vi "Bool_array_to_digital_waveform.vi"(0 "Olfactormeter parameters":T1, 1 "Type":string, 2 "odour waveform array":bool[](array[boolean]), 4 "i":i32) -> (6 "digital waveform":digitalwaveform(waveform))   [LabVIEW 2016]
uses:
  <vilib>/Waveform/DWDTOps.llb/DWDT Boolean Array to Digital.vi
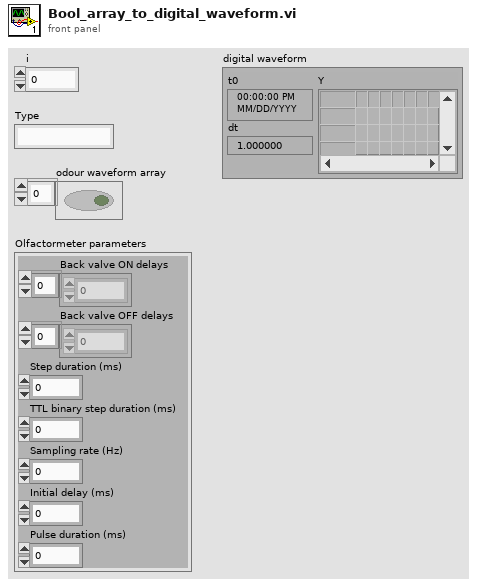
[diagram p1: front panel]
types:
  T1 = cluster{"Back valve ON delays":dbl[], "Back valve OFF delays":dbl[], "Step duration (ms)":dbl, "TTL binary step duration (ms)":dbl, "Sampling rate (Hz)":dbl, "Initial delay (ms)":dbl, "Pulse duration (ms)":dbl}
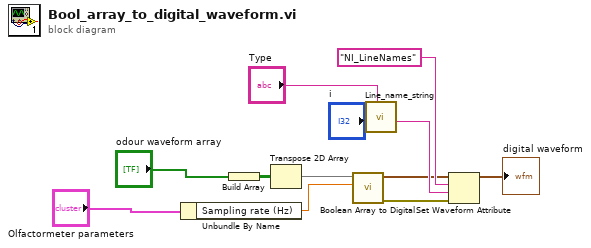
[diagram p0: block diagram]
diagram:
  n1 = Unbundle By Name("Olfactormeter parameters") -> ("Sampling rate (Hz)"=w11:dbl)
  n2 = Build Array("odour waveform array") -> (w8:bool[][])
  n3 = Transpose 2D Array(2D array=w8) -> (transposed array=w9:bool[][])
  n4 = call-poly <vilib>:"Boolean Array to Digital.vi"("sample rate"=w11, "boolean array"=w9) -> ("error out"=w12:errorcluster, "digital waveform"=w2:digitalwaveform)  [unwired: 8 in]
  n5 = call "Line_name_string.vi"("Type"="Type", "i"="i") -> ("name out"=w5:string)  [unwired: 9 in]
  n6 = Set Waveform Attribute(4:w12, 5:w5, 6:"NI_LineNames" ("name"), 7:w2) -> (3:→"digital waveform":digitalwaveform)  [unwired: 2 out]
